vi "Update WebSocket Clients.vi"(9 "Initialize":bool, 10 "delta JSON":string) -> ()   [LabVIEW 2019]
uses:
  <vilib>/MediaMongrels Ltd/WebSockets/WebSockets/WebSocket/WebSocket.lvclass
panel:
  out "Clients":i32
  out "Sent":cluster{"deltaT":u32, "buffer":string}[](array[cluster])
  in  "Trace":bool
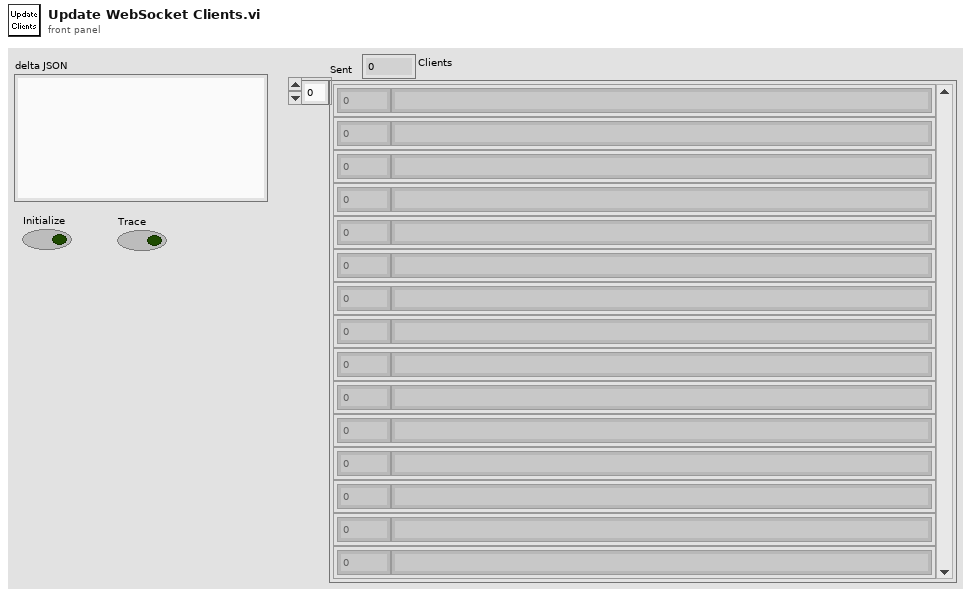
[diagram p1: front panel]
types:
  T1 = enum16{"add client", "remove client", "get clients", "clear"}
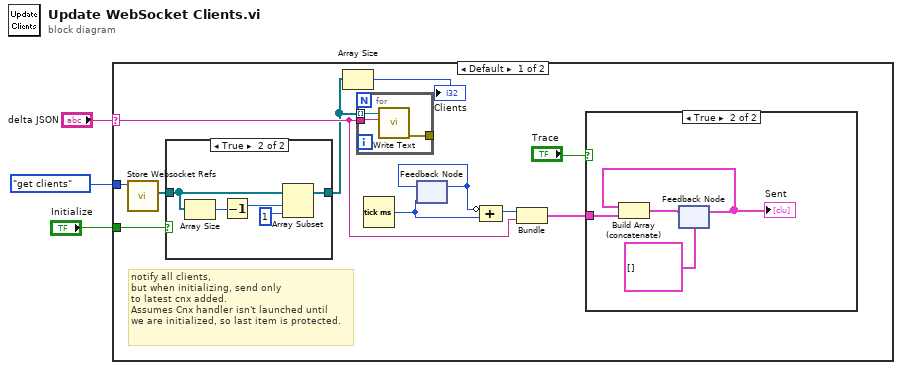
[diagram p0: block diagram]
diagram:
  n1 = case shown="Default" "delta JSON" {
    selector: "delta JSON" -> [w8 _]
    tunnel: T1."get clients" ("menu") -> [w14 _]
    tunnel: "Initialize" -> [w13 _]
    frame Default {
      # "notify all clients,\nbut when initializing, send only\nto latest cnx added.\nAssumes Cnx handler isn't launched until\nwe are initialized, so last item is protected."
      n2 = call "Store Websocket Refs.vi"("menu"=w14) -> ("Clients"=w12:refnum<class "WebSocket.lvclass">[])  [unwired: 10 in]
      n3 = case shown="True" w13 {
        tunnel: w12 -> [w19 w22]
        tunnel: [w19 w24] -> w7
        frame False {
        }
        frame True {
          n4 = Array Size(array=w22) -> (size(s)=w21:i32)
          n5 = Decrement(x=w21) -> (x-1=w20:i32)
          n6 = Array Subset(array=w22, index=w20, length=1) -> (w24:refnum<class "WebSocket.lvclass">[])
        }
      }
      n7 = Array Size(array=w7) -> (size(s)=→"Clients":i32)
      n8 = for {
        tunnel: w8 -> [w27]
        tunnel: w7 -> [w26] mode=indexing
        tunnel: [w25] -> _
        n9 = call-dynamic "Write Text.vi"("String Data"=w27, "WebSocket in"=w26) -> ("error out"=w25:errorcluster)  [unwired: 8 in, 1 out]
      }
      n10 = Tick Count (ms)() -> (millisecond timer value=w11:u32)
      n11 = feedback #1(w11) -> (w10:u32)
      n12 = feedback-in #1(w10) -> ()
      n13 = Compound Arithmetic op=ADD(invert w10, w11) -> (w9:u32)
      n14 = Bundle(w9, w8) -> (w4:cluster{u32, string})  [unwired: 1 in]
      n15 = case shown="True" "Trace" {
        tunnel: w4 -> [_ w18]
        frame False {
        }
        frame True {
          n16 = feedback #2(cluster{u32, string}[] []) -> (w16:cluster{u32, string}[])
          "Sent" <- w16
          n17 = Build Array (concatenate)(w16, w18) -> (w17:cluster{u32, string}[])
          n18 = feedback-in #2(w17) -> ()
        }
      }
    }
    frame "" {
      # "server received\nthis from a client"
    }
  }
